vi "GDSString_FindTextBasedCodeDocumenation.vi"(0 "Text":string="\n   private String name;\n   private String dept;\n   private int salary;\n   private List<Employee> subordinates;\n\n   // constructor\n   public Employee(String name,String dept, int sal) ", 1 "StringStartOffset(Default=-1 => 0 for Forward, StrLenght for Backwards)":i32=-1, 2 "Search Backwards":bool, 4 "CommentHasToBeTheFirstItem(True)":bool=TRUE, 5 "error in (no error)":errorcluster) -> (14 "Document":string="constructor", 15 "Found":bool=TRUE, 17 "IndexBeforeDocument(Or after when searching Backwards)":i32=102, 18 "IndexAfterDocument(Or before when searching Backwards)":i32=119, 19 "error out":errorcluster)   [LabVIEW 2020]
doc: "Finds Java or c# comments\n/***\n* JAVA\n**/\n/// <C#-XML>\n/// </C#-XML>"
uses:
  <vilib>/regexp/Match Regular Expression.xnode
panel:
  out "substring before match":string
  out "After":string="constructor"
  out "Before":string="constructor"
  # "119"
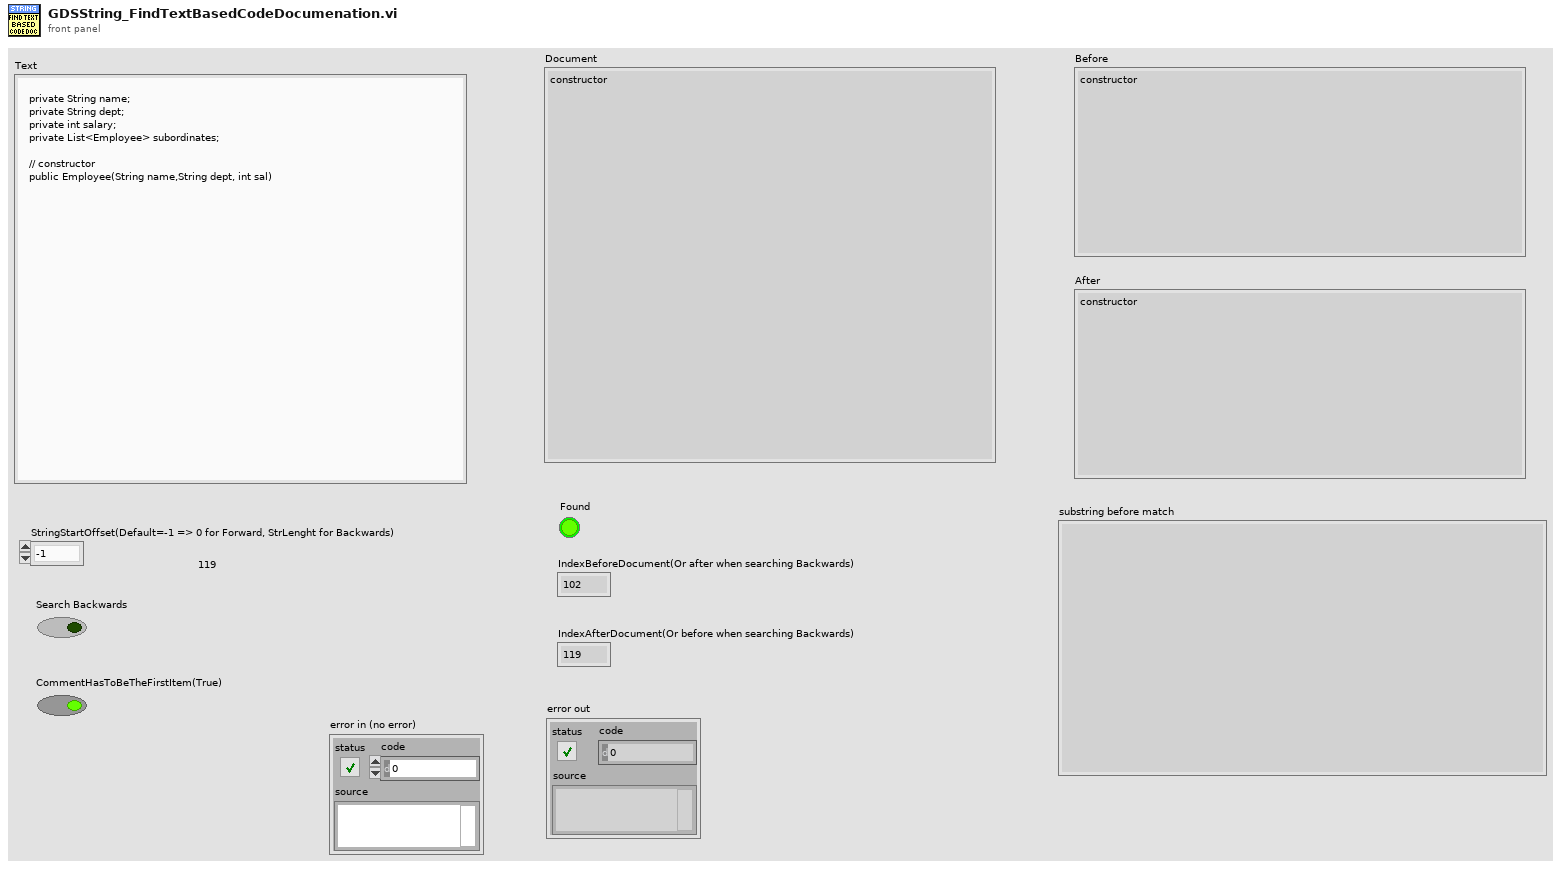
[diagram p1: front panel]
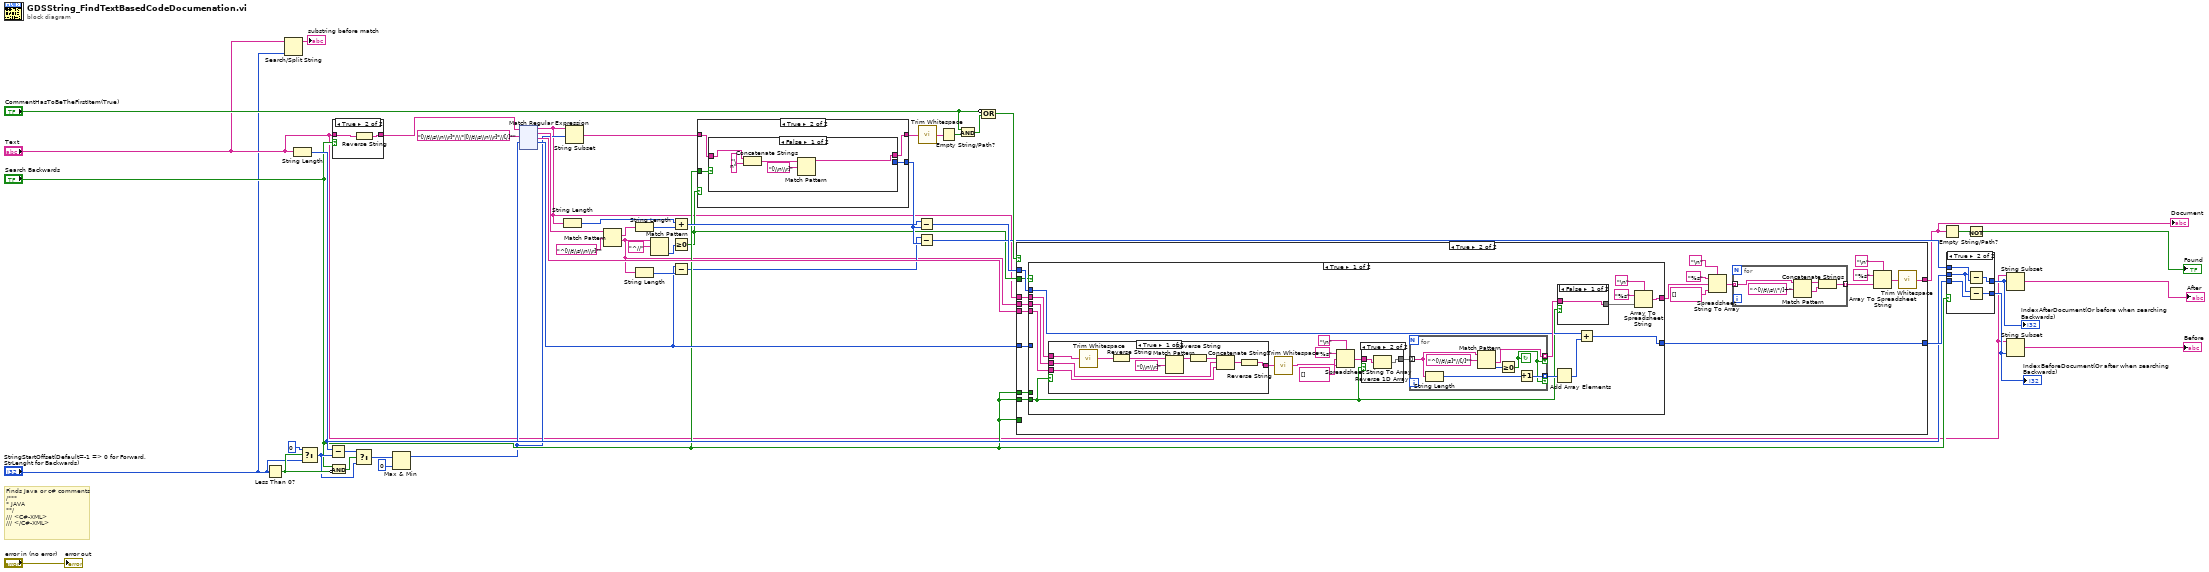
[diagram p0: block diagram]
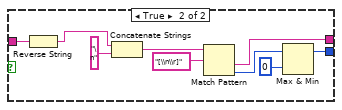
[diagram p3: hidden frame]
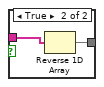
[diagram p6: hidden frame]
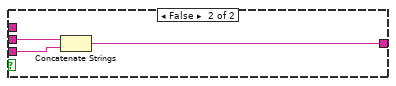
[diagram p8: hidden frame]
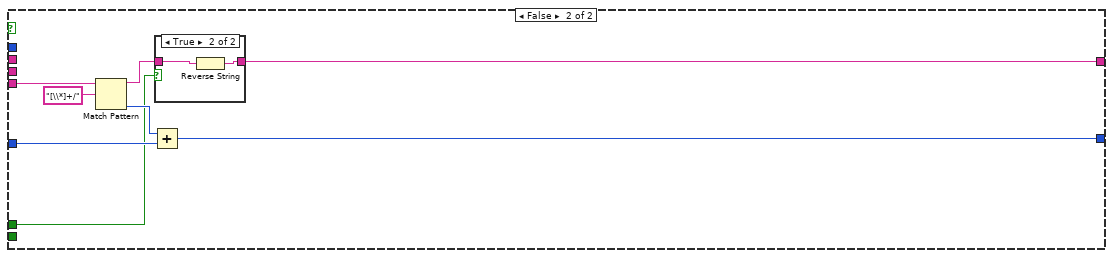
[diagram p9: hidden frame]
diagram:
  # "Finds Java or c# comments\n/***\n* JAVA\n**/\n/// <C#-XML>\n/// </C#-XML>"
  n1 = Less Than 0?(x="StringStartOffset(Default=-1 => 0 for Forward, StrLenght for Backwards)") -> (x < 0?=w42:bool)
  n2 = Search/Split String(string="Text", offset (0)="StringStartOffset(Default=-1 => 0 for Forward, StrLenght for Backwards)") -> (substring before match=→"substring before match":string)  [unwired: 1 in, 2 out]
  n3 = String Length(string="Text") -> (length=w21:i32)
  n4 = Select(t=0, s=w42, f="StringStartOffset(Default=-1 => 0 for Forward, StrLenght for Backwards)") -> (s? t:f=w40:i32)
  n5 = Subtract(x=w21, y=w40) -> (x-y=w39:i32)
  n6 = case shown="True" "Search Backwards" {
    tunnel: "Text" -> [w50 w52]
    tunnel: [w50 w51] -> w31
    frame False {
    }
    frame True {
      n7 = Reverse String(1:w52) -> (0:w51:string)
    }
  }
  n8 = Compound Arithmetic op=AND("Search Backwards", invert w42) -> (w41:bool)
  n9 = Select(t=w39, s=w41, f=w40) -> (s? t:f=w38:i32)
  n10 = Max & Min(x=w38, y=0 ("t")) -> (max(x,y)=w15:i32)  [unwired: 1 out]
  n11 = xnode "Match Regular Expression"("input string"=w31, "regular expression"="[\\t\\s\\n\\r]*/\\*|[\\t\\s\\n\\r]*//[/]*", "offset (0)"=w15) -> ("before match"=w9:string, "whole match"=w30:string, "after match"=w48:string, "offset past match"=w33:i32)  [unwired: 3 in, 1 out]
  n12 = String Length(string=w9) -> (length=w28:i32)
  n13 = String Subset(string=w9, offset (0)=w15) -> (substring=w10:string)  [unwired: 1 in]
  n14 = Match Pattern(string=w30, regular expression="^[\\t\\s\\n\\r]*") -> (match substring=w25:string, after substring=w14:string)  [unwired: 1 in, 2 out]
  n15 = String Length(string=w25) -> (length=w27:i32)
  n16 = String Length(string=w14) -> (length=w34:i32)
  n17 = Match Pattern(string=w14, regular expression="^//") -> (offset past match=w12:i32)  [unwired: 1 in, 3 out]
  n18 = Add(x=w28, y=w27) -> (x+y=w26:i32)
  n19 = Greater Or Equal To 0?(x=w12) -> (x >= 0?=w11:bool)
  n20 = Subtract(x=w33, y=w34) -> (x-y=w17:i32)
  n21 = case shown="True" w11 {
    tunnel: [w53 w56] -> w24
    tunnel: "Search Backwards" -> [_ w57]
    tunnel: w10 -> [w53 w55]
    tunnel: [_ w54] -> w18
    frame False {
    }
    frame True {
      n22 = case shown="False" w57 {
        tunnel: w55 -> [w59 w71]
        tunnel: [w61 w68] -> w56
        tunnel: [_ w66] -> w54
        frame False {
          n23 = Concatenate Strings(w59, "\n" ("string")) -> (w58:string)
          n24 = Match Pattern(string=w58, regular expression="[\\n\\r]") -> (before substring=w61:string)  [unwired: 1 in, 3 out]
        }
        frame True {
          n25 = Reverse String(1:w71) -> (0:w70:string)
          n26 = Concatenate Strings(w70, "\n" ("string")) -> (w64:string)
          n27 = Match Pattern(string=w64, regular expression="[\\n\\r]") -> (after substring=w68:string, offset past match=w67:i32)  [unwired: 1 in, 2 out]
          n28 = Max & Min(x=w67, y=0) -> (max(x,y)=w66:i32)  [unwired: 1 out]
        }
      }
    }
  }
  n29 = Subtract(x=w26, y=w18) -> (x-y=w19:i32)
  n30 = Subtract(x=w17, y=w18) -> (x-y=w16:i32)
  n31 = call <vilib>:"Trim Whitespace.vi"("string"=w24) -> ("trimmed string"=w23:string)  [unwired: 1 in]
  n32 = Empty String/Path?(string/path=w23) -> (empty?=w22:bool)
  n33 = And(x="CommentHasToBeTheFirstItem(True)", y=w22) -> (x .and. y?=w44:bool)
  n34 = Compound Arithmetic op=OR(invert "CommentHasToBeTheFirstItem(True)", w44) -> (w43:bool)
  n35 = case shown="True" w43 {
    tunnel: w48 -> [_ w76]
    tunnel: w14 -> [_ w82]
    tunnel: [_ w81] -> w8
    tunnel: "Search Backwards" -> [_ _]
    tunnel: w33 -> [_ w80]
    tunnel: [_ w79] -> w32
    tunnel: w19 -> [_ w78]
    tunnel: "Search Backwards" -> [_ w75]
    tunnel: "Search Backwards" -> [_ w74]
    tunnel: w9 -> [_ w73]
    tunnel: w11 -> [_ w72]
    frame False {
    }
    frame True {
      n36 = case shown="True" w72 {
        tunnel: [w102 w138] -> w77
        tunnel: w76 -> [w96 w143]
        tunnel: w80 -> [_ w141]
        tunnel: [w99 w140] -> w79
        tunnel: w78 -> [w98 _]
        tunnel: w75 -> [_ w137]
        tunnel: w74 -> [w91 _]
        tunnel: w73 -> [w95 _]
        tunnel: w82 -> [w97 _]
        frame True {
          n37 = case shown="True" w91 {
            tunnel: [w123 w129] -> w108
            tunnel: w97 -> [w125 w128]
            tunnel: w96 -> [w124 w127]
            tunnel: w95 -> [w122 _]
            frame True {
              n38 = call <vilib>:"Trim Whitespace.vi"("string"=w122) -> ("trimmed string"=w120:string)  [unwired: 1 in]
              n39 = Reverse String(1:w120) -> (0:w119:string)
              n40 = Match Pattern(string=w119, regular expression="[\\n\\r]") -> (before substring=w118:string)  [unwired: 1 in, 3 out]
              n41 = Reverse String(1:w118) -> (0:w117:string)
              n42 = Concatenate Strings(w117, w125, w124) -> (w126:string)
              n43 = Reverse String(1:w126) -> (0:w123:string)
            }
            frame False {
              n44 = Concatenate Strings(w128, w127) -> (w129:string)
            }
          }
          n45 = call <vilib>:"Trim Whitespace.vi"("string"=w108) -> ("trimmed string"=w94:string)  [unwired: 1 in]
          n46 = Spreadsheet String To Array(delimiter (Tab)="\n", format string="%s", spreadsheet string=w94, array type (2D Dbl)=string[] []) -> (array=w106:string[])
          n47 = case shown="True" w91 {
            tunnel: w106 -> [w114 w116]
            tunnel: [w114 w115] -> w92
            frame False {
            }
            frame True {
              n48 = Reverse 1D Array(array=w116) -> (reversed array=w115:string[])
            }
          }
          n49 = for {
            tunnel: w92 -> [w133] mode=indexing
            tunnel: [w135] -> w103 mode=indexing if=w130
            tunnel: [w131] -> w101 mode=indexing if=w130
            stop <- w130 continue-if-true
            n50 = String Length(string=w133) -> (length=w132:i32)
            n51 = Match Pattern(string=w133, regular expression="^[\\t\\s]*//[/]*") -> (after substring=w135:string, offset past match=w134:i32)  [unwired: 1 in, 2 out]
            n52 = Greater Or Equal To 0?(x=w134) -> (x >= 0?=w130:bool)
            n53 = Increment(x=w132) -> (x+1=w131:i32)
          }
          n54 = Add Array Elements(numeric array=w101) -> (sum=w100:i32)
          n55 = case shown="False" w91 {
            tunnel: w103 -> [w111 w113]
            tunnel: [w111 w112] -> w93
            frame False {
            }
            frame True {
              n56 = Reverse 1D Array(array=w113) -> (reversed array=w112:string[])
            }
          }
          n57 = Add(x=w98, y=w100) -> (x+y=w99:i32)
          n58 = Array To Spreadsheet String(delimiter (Tab)="\n", array=w93, 3:"%s" ("format string")) -> (spreadsheet string=w102:string)
        }
        frame False {
          n59 = Match Pattern(string=w143, regular expression="[\\*]+/") -> (before substring=w139:string, offset past match=w142:i32)  [unwired: 1 in, 2 out]
          n60 = Add(x=w142, y=w141) -> (x+y=w140:i32)
          n61 = case shown="True" w137 {
            tunnel: w139 -> [w145 w147]
            tunnel: [w145 w146] -> w138
            frame False {
            }
            frame True {
              n62 = Reverse String(1:w147) -> (0:w146:string)
            }
          }
        }
      }
      n63 = Spreadsheet String To Array(delimiter (Tab)="\n", format string="%s", spreadsheet string=w77, array type (2D Dbl)=string[] []) -> (array=w87:string[])
      n64 = for {
        tunnel: w87 -> [w152] mode=indexing
        tunnel: [w148] -> w86 mode=indexing
        n65 = Match Pattern(string=w152, regular expression="^[\\t\\s\\*/]+") -> (before substring=w150:string, after substring=w149:string)  [unwired: 1 in, 2 out]
        n66 = Concatenate Strings(w150, w149) -> (w148:string)
      }
      n67 = Array To Spreadsheet String(delimiter (Tab)="\n", array=w86, 3:"%s" ("format string")) -> (spreadsheet string=w83:string)
      n68 = call <vilib>:"Trim Whitespace.vi"("string"=w83) -> ("trimmed string"=w81:string)  [unwired: 1 in]
    }
  }
  "Document" <- w8
  n69 = Empty String/Path?(string/path=w8) -> (empty?=w46:bool)
  n70 = case shown="True" "Search Backwards" {
    tunnel: w16 -> [w154 w159]
    tunnel: [w154 w155] -> w5
    tunnel: [w153 w158] -> w7
    tunnel: w32 -> [w153 w156]
    tunnel: w21 -> [_ w157]
    frame False {
    }
    frame True {
      n71 = Subtract(x=w157, y=w159) -> (x-y=w158:i32)
      n72 = Subtract(x=w157, y=w156) -> (x-y=w155:i32)
    }
  }
  "IndexAfterDocument(Or before when searching Backwards)" <- w7
  "IndexBeforeDocument(Or after when searching Backwards)" <- w5
  n73 = Not(x=w46) -> (.not. x?=→"Found":bool)
  n74 = String Subset(string="Text", offset (0)=w7) -> (substring=→"After":string)  [unwired: 1 in]
  n75 = String Subset(string="Text", length (rest)=w5) -> (substring=→"Before":string)  [unwired: 1 in]
  "error out" <- "error in (no error)"
